vi "Enable Burner Cycle.vi"(8 "error in (no error)":errorcluster, 11 "Data Cluster In":T1 {"VestaTemperature"."Water Heater Temp (°F)" min=32 max=203}) -> (0 "error out":errorcluster, 1 "Send_Vesta_Message":u8, 3 "Data Cluster Output":T1 {"VestaTemperature"."Water Heater Temp (°F)" min=32 max=203})   [LabVIEW 2023]
uses:
  Drivers/Resideo Gas Valve/Type Definitions/Temperature Control.ctl
  Message Queue/Message Queue.lvlib
  Message Queue/Enqueue Message (Single).vi
  Drivers/Resideo Gas Valve/Type Definitions/Vesta Info.ctl
  controls/Burner Duty Cycle.ctl
  controls/Timer Application Cluster.ctl
  controls/UI Data.ctl
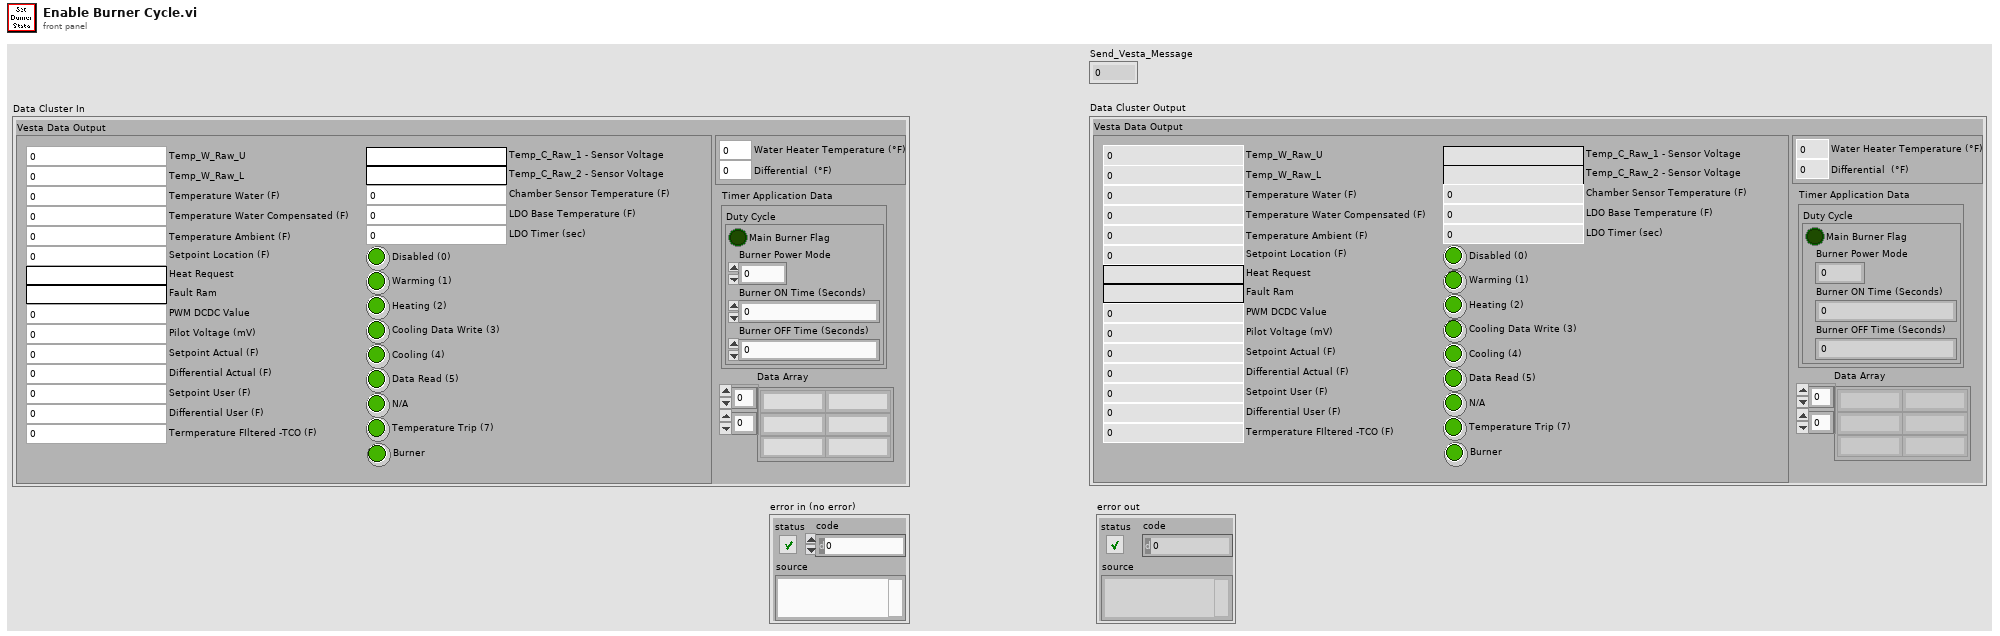
[diagram p1: front panel]
types:
  T1 = typedef "UI Data.ctl" = cluster{"Vesta Data Output":T2, "VestaTemperature":T3, "Timer Application Data":T4, "Data Array":string[][]}
  T2 = typedef "Vesta Info.ctl" = cluster{"Temp_W_Raw_U":u16, "Temp_W_Raw_L":u16, "Temperature Water (F)":dbl, "Temperature Water Compensated (F)":dbl, "Temperature Ambient (F)":dbl, "Setpoint Location (F)":dbl, "Heat Request":string, "Fault Ram":string, "PWM DCDC Value":u16, "Pilot Voltage (mV)":dbl, "Setpoint Actual (F)":dbl, "Differential Actual (F)":dbl, "Setpoint User (F)":dbl, "Differential User (F)":dbl, "Termperature FIltered -TCO (F)":dbl, "Temp_C_Raw_1 - Sensor Voltage":string, "Temp_C_Raw_2 - Sensor Voltage":string, "Chamber Sensor Temperature (F)":dbl, "LDO Base Temperature (F)":dbl, "LDO Timer (sec)":i16, "Disabled (0)":bool, "Warming (1)":bool, "Heating (2)":bool, "Cooling Data Write (3)":bool, "Cooling (4)":bool, "Data Read (5)":bool, "N/A":bool, "Temperature Trip (7)":bool, "Burner":bool}
  T3 = typedef "Temperature Control.ctl" = cluster{"Water Heater Temp (°F)":u16, "Differential  (°F)":dbl}
  T4 = typedef "Timer Application Cluster.ctl" = cluster{"Duty Cycle":T5}
  T5 = typedef "Burner Duty Cycle.ctl" = cluster{"Burner ON Time (Seconds)":dbl, "Burner OFF Time (Seconds)":dbl, "Main Burner Flag":bool, "Burner Power Mode":u8}
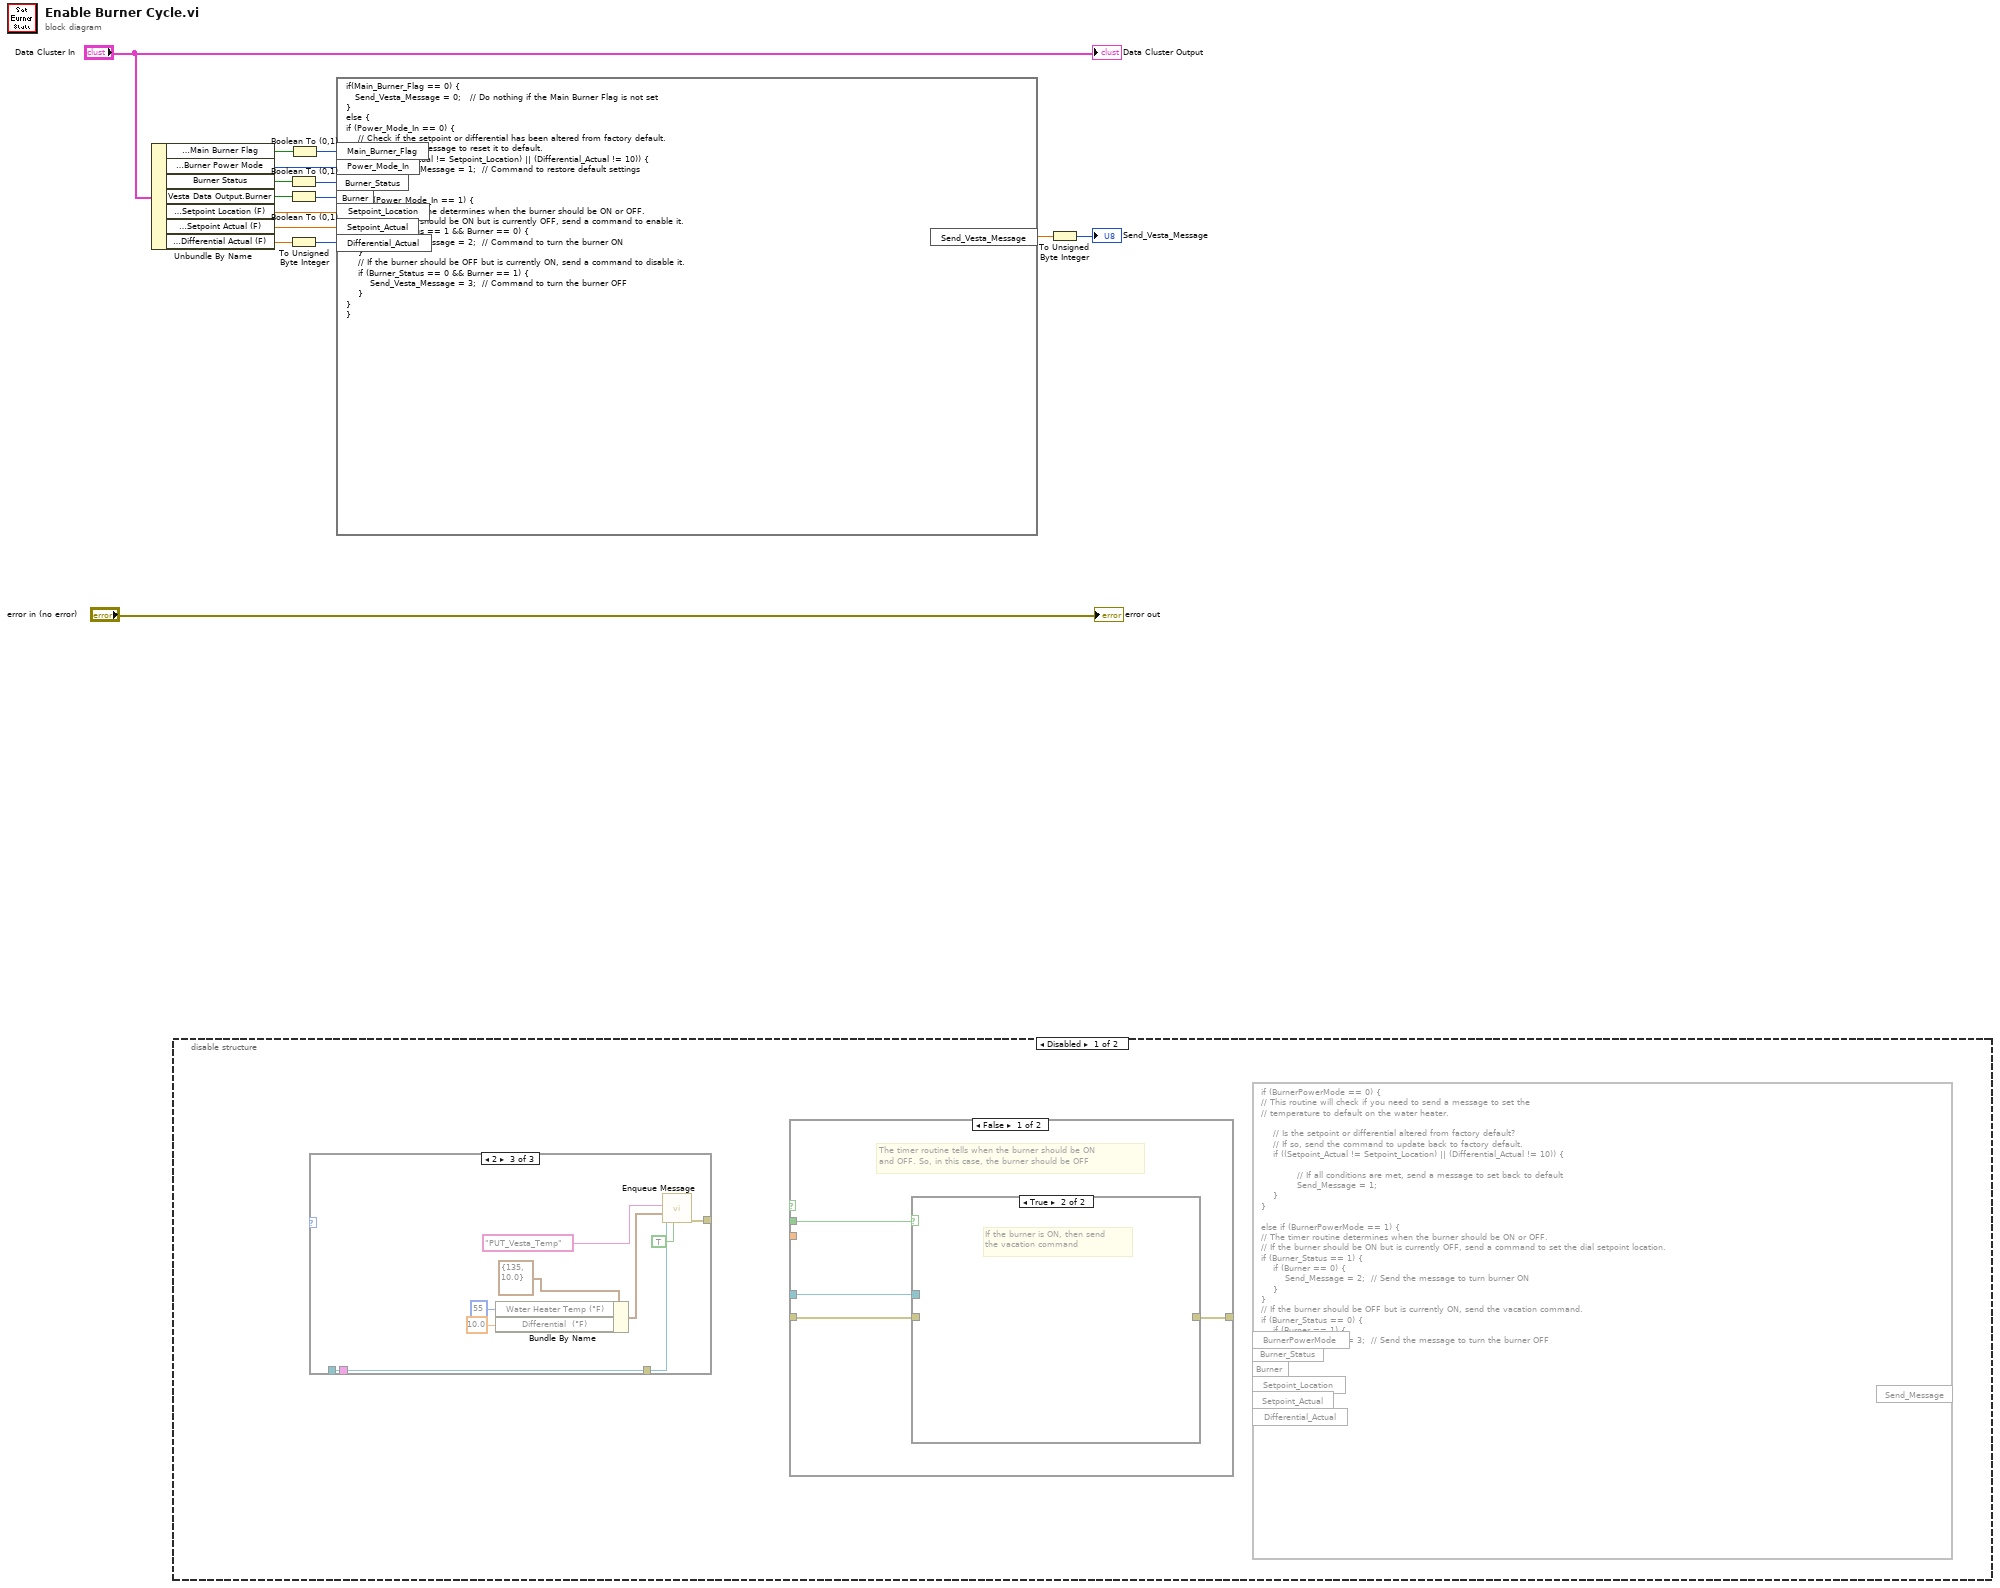
[diagram p0: block diagram]
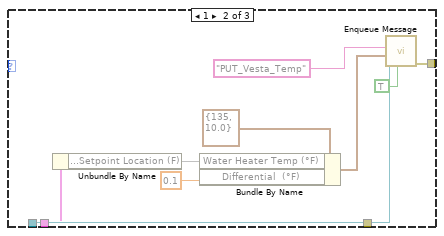
[diagram p3: hidden frame]
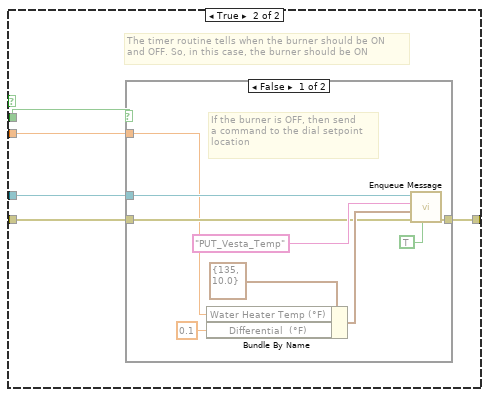
[diagram p5: hidden frame]
diagram:
  n1 = Unbundle By Name("Data Cluster In") -> ("Timer Application Data.Duty Cycle.Main Burner Flag"=w2:bool, "Timer Application Data.Duty Cycle.Burner Power Mode"=w6:u8, "Burner Status"=w14:bool, "Vesta Data Output.Burner"=w13:bool, "Vesta Data Output.Setpoint Location (F)"=w8:dbl, "Vesta Data Output.Setpoint Actual (F)"=w7:dbl, "Vesta Data Output.Differential Actual (F)"=w9:dbl)
  n2 = disable-structure shown="Disabled" {
    frame Disabled {
      n3 = case shown="2" {
        selector: _ -> [_ _ _]
        tunnel: _ -> [_ w21 w29]
        tunnel: _ -> [w16 w20 w28]
        tunnel: _ -> [_ w19 _]
        tunnel: [w16 w17 w27] -> _
        frame 0, Default {
          # "Do nothing. All is good."
        }
        frame 1 {
          n4 = Unbundle By Name(w19) -> ("Vesta Data Output.Setpoint Location (F)"=w18)
          n5 = Bundle By Name(cluster=T3 {"Water Heater Temp (°F)"=135, "Differential  (°F)"=10.0} ("VestaTemperature"), "Water Heater Temp (°F)"=w18, "Differential  (°F)"=0.1) -> (w26:T3)
          n6 = call-poly "Enqueue Message.vi"("Priority Message? (F)"=TRUE, "error in (no error)"=w20, "Message Data"=w26, "Message"="PUT_Vesta_Temp", "Message Queue"=w21) -> ("error out"=w17:errorcluster)  [unwired: 5 in, 1 out]
        }
        frame 2 {
          n7 = Bundle By Name(cluster=T3 {"Water Heater Temp (°F)"=135, "Differential  (°F)"=10.0} ("VestaTemperature"), "Water Heater Temp (°F)"=u16 55, "Differential  (°F)"=10.0) -> (w33:T3)
          n8 = call-poly "Enqueue Message.vi"("Priority Message? (F)"=TRUE, "error in (no error)"=w28, "Message Data"=w33, "Message"="PUT_Vesta_Temp", "Message Queue"=w29) -> ("error out"=w27:errorcluster)  [unwired: 5 in, 1 out]
        }
      }
      n9 = case shown="False" {
        selector: _ -> [_ _]
        tunnel: _ -> [w39 w43]
        tunnel: [w38 w45] -> _
        tunnel: _ -> [w37 w44]
        tunnel: _ -> [w36 w41]
        tunnel: _ -> [_ w42]
        frame False {
          # "The timer routine tells when the burner should be ON\nand OFF. So, in this case, the burner should be OFF"
          n10 = case shown="True" w36 {
            tunnel: w39 -> [_ _]
            tunnel: [w40 _] -> w38
            tunnel: w37 -> [w40 _]
            frame False {
              # "If the burner is OFF, no \nneed to send a command."
            }
            frame True {
              # "If the burner is ON, then send\nthe vacation command"
            }
          }
        }
        frame True {
          # "The timer routine tells when the burner should be ON\nand OFF. So, in this case, the burner should be ON"
          n11 = case shown="False" w41 {
            tunnel: [w49 w55] -> w45
            tunnel: w44 -> [w48 w55]
            tunnel: w43 -> [w47 _]
            tunnel: w42 -> [w46 _]
            frame False {
              # "If the burner is OFF, then send\na command to the dial setpoint\nlocation"
              n12 = Bundle By Name(cluster=T3 {"Water Heater Temp (°F)"=135, "Differential  (°F)"=10.0} ("VestaTemperature"), "Water Heater Temp (°F)"=w46, "Differential  (°F)"=0.1) -> (w54:T3)
              n13 = call-poly "Enqueue Message.vi"("Priority Message? (F)"=TRUE, "error in (no error)"=w48, "Message Data"=w54, "Message"="PUT_Vesta_Temp", "Message Queue"=w47) -> ("error out"=w49:errorcluster)  [unwired: 5 in, 1 out]
            }
            frame True {
              # "If the burner is ON, no \nneed to send a command."
            }
          }
        }
      }
      n14 = formula code="if (BurnerPowerMode == 0) {\n// This routine will check if you need to send a message to set the \n// temperature to default on the water heater.\n    \n    // Is the setpoint or differential altered from factory default?\n    // If so, send the command to update back to factory default.\n    if ((Setpoint_Actual != Setpoint_Location) || (Differential_Actual != 10)) {             \n            \n            // If all conditions are met, send a message to set back to default\n            Send_Message = 1;  \n    }\n}\n\nelse if (BurnerPowerMode == 1) {\n// The timer routine determines when the burner should be ON or OFF.\n// If the burner should be ON but is currently OFF, send a command to set the dial setpoint location.\nif (Burner_Status == 1) {  \n    if (Burner == 0) {  \n        Send_Message = 2;  // Send the message to turn burner ON\n    }\n}\n// If the burner should be OFF but is currently ON, send the vacation command.\nif (Burner_Status == 0) {  \n    if (Burner == 1) {  \n        Send_Message = 3;  // Send the message to turn the burner OFF\n    }\n}\n}"() -> ()  [unwired: 6 in, 1 out]
    }
    frame Enabled {
    }
  }
  n15 = Boolean To (0,1)(Boolean=w14) -> (0, 1=w12:i16)
  n16 = Boolean To (0,1)(Boolean=w13) -> (0, 1=w11:i16)
  n17 = To Unsigned Byte Integer(number=w9) -> (unsigned 8bit integer=w10:u8)
  n18 = Boolean To (0,1)(Boolean=w2) -> (0, 1=w1:i16)
  n19 = formula code="if(Main_Burner_Flag == 0) {\n   Send_Vesta_Message = 0;   // Do nothing if the Main Burner Flag is not set\n}\nelse {\nif (Power_Mode_In == 0) {\n    // Check if the setpoint or differential has been altered from factory default.\n    // If so, send a message to reset it to default.\n    if ((Setpoint_Actual != Setpoint_Location) || (Differential_Actual != 10)) {  \n        Send_Vesta_Message = 1;  // Command to restore default settings\n    }\n} \nelse if (Power_Mode_In == 1) {\n    // The timer routine determines when the burner should be ON or OFF.\n    // If the burner should be ON but is currently OFF, send a command to enable it.\n    if (Burner_Status == 1 && Burner == 0) {  \n        Send_Vesta_Message = 2;  // Command to turn the burner ON\n    }\n    // If the burner should be OFF but is currently ON, send a command to disable it.\n    if (Burner_Status == 0 && Burner == 1) {  \n        Send_Vesta_Message = 3;  // Command to turn the burner OFF\n    }\n}\n}"("Burner"=w11, "Burner_Status"=w12, "Setpoint_Location"=w8, "Setpoint_Actual"=w7, "Differential_Actual"=w10, "Power_Mode_In"=w6, "Main_Burner_Flag"=w1) -> ("Send_Vesta_Message"=w15:dbl)
  n20 = To Unsigned Byte Integer(number=w15) -> (unsigned 8bit integer=→"Send_Vesta_Message":u8)
  "error out" <- "error in (no error)"
  "Data Cluster Output" <- "Data Cluster In"
